vi "Live ROI Information Display.vi"(0 "Event Type":T1=enum."Value Change", 2 "ROI Mask REF":T2, 11 "IMAQ Image Display Ref":refnum<vi>) -> ()   [LabVIEW 2016]
uses:
  <vilib>/vision/Image Controls.llb/IMAQ Image.ctl
  <vilib>/event_ctls.llb/lveventtype.ctl
  Hardware Configuration/Hardware Configuration Controls/Standard Action.ctl
  <vilib>/vision/NI_Vision_Development_Module.lvlib
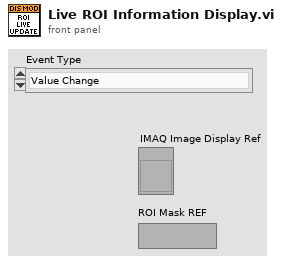
[diagram p1: front panel]
types:
  T1 = typedef "lveventtype.ctl" = enum32{"Null", "Timeout", "Annotation Menu Selection", "Annotation Menu Selection?", "App Instance Close", "App Instance Close?", "Autoscale Range Change", "Bookmark Info Change", "Cell Edit", "Cell Edit?", "Cursor Grab", "Cursor Grab?", "Cursor Menu Selection", "Cursor Menu Selection?", "Cursor Move", "Cursor Release", "Data Change", "Direction Change", "Display State Change", "Drag Ended", "Drag Enter", "Drag Leave", "Drag Over", "Drag Source Update", "Drag Starting", "Drag Starting?", "Drop", "Exec State Change", "Key Down", "Key Down?", "Key Repeat", "Key Repeat?", "Key Up", "Listbox Double Click", "Menu Activation?", "Menu Selection (App)", "Menu Selection? (App)", "Menu Selection (User)", "Mouse Down", "Mouse Down?", "Mouse Enter", "Mouse Leave", "Mouse Move", "Mouse Up", "Mouse Wheel", "NI Security User Change (App)", "Pane Size", "Panel Close", "Panel Close?", "Panel Resize", "Plot Attribute Change", "Scale Range Change", "Shortcut Menu Activation?", "Shortcut Menu Selection (App)", "Shortcut Menu Selection? (App)", "Shortcut Menu Selection (User)", "Tree Double Click", "Tree Drag", "Tree Drag?", "Tree Drop", "Tree Drop?", "Tree Item Close", "Tree Item Close?", "Tree Item Open", "Tree Item Open?", "User Event", "Value Change"}
  T2 = typedef "IMAQ Image.ctl" = refnum<image>
  T3 = typedef "Standard Action.ctl" = enum16{"Read", "Write"}
  T4 = cluster{"Global Rectangle":i32[], "Contours":cluster{"Contour Type":u32, "ROI Type":u32, "Points":i32[]}[]}
  T5 = cluster{"Contour Type":u32, "ROI Type":u32, "Points":i32[]}[]
  T6 = cluster{"Contour Type":u32, "ROI Type":u32, "Points":i32[]}
  T7 = cluster{"Mean Value":sgl, "Standard Variation":sgl, "Minimal Value":sgl, "Maximal Value":sgl, "Area (calibrated)":sgl, "Area (pixels)":u32, "%":sgl, "Calibration Valid":bool}
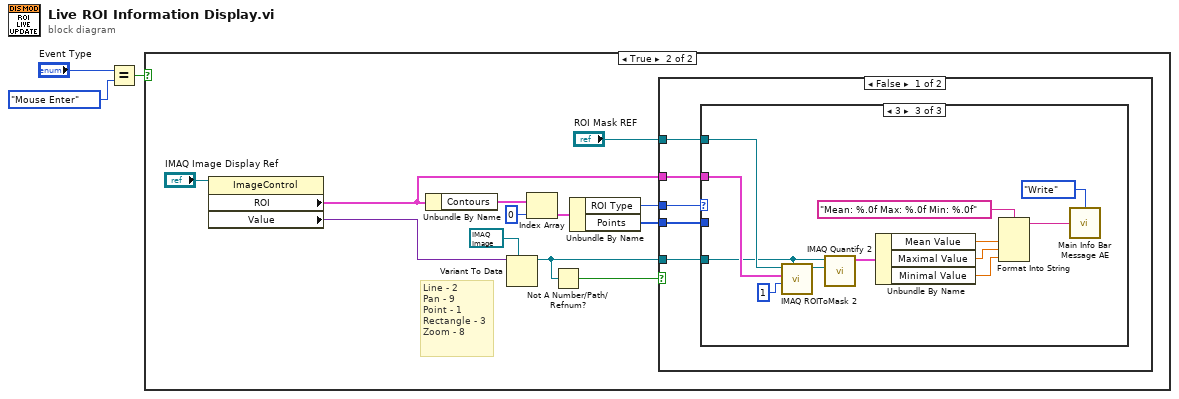
[diagram p0: block diagram]
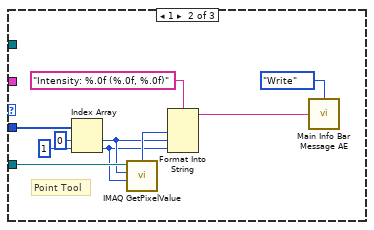
[diagram p4: hidden frame]
diagram:
  n1 = Equal?(x="Event Type", y=lveventtype."Mouse Enter") -> (x = y?=w1:bool)
  n2 = case shown="True" w1 {
    frame False {
    }
    frame True {
      # "Line - 2\nPan - 9\nPoint - 1\nRectangle - 3\nZoom - 8"
      n3 = property class="ImageControl"(reference="IMAQ Image Display Ref") -> ("ROI"=w9:T4, "Value"=w8:variant)  [unwired: 1 in, 2 out]
      n4 = Unbundle By Name(w9) -> ("Contours"=w14:T5)
      n5 = Variant To Data(type=T2 refnum ("New Image"), Variant=w8) -> (data=w6:T2)  [unwired: 1 in, 1 out]
      n6 = Index Array(array=w14, index=0) -> (element=w12:T6)
      n7 = Not A Number/Path/Refnum?(number/path/refnum=w6) -> (NaN/Path/Refnum?=w5:bool)
      n8 = Unbundle By Name(w12) -> ("ROI Type"=w11:u32, "Points"=w10:i32[])
      n9 = case shown="False" w5 {
        tunnel: w11 -> [w20 _]
        tunnel: w10 -> [w19 _]
        tunnel: w9 -> [w18 _]
        tunnel: "ROI Mask REF" -> [w17 _]
        tunnel: w6 -> [w16 _]
        frame False {
          n10 = case shown="3" w20 {
            tunnel: w19 -> [_ w30 _]
            tunnel: w18 -> [_ _ w42]
            tunnel: w17 -> [_ _ w41]
            tunnel: w16 -> [_ w26 w40]
            frame Default {
            }
            frame 1 {
              # "Point Tool"
              n11 = Index Array(array=w30, index #1=0 ("index"), index #2=1 ("index")) -> (element #1=w24:i32, element #2=w23:i32)
              n12 = call "IMAQ GetPixelValue"("Image"=w26, "X Coordinate"=w24, "Y Coordinate"=w23) -> ("Pixel Value (U16)"=w27:u16)  [unwired: 3 in, 4 out]
              n13 = Format Into String(format string="Intensity: %.0f (%.0f, %.0f)", w27, w24, w23) -> (resulting string=w22:string)  [unwired: 2 in, 1 out]
              n14 = call "Main Info Bar Message AE.vi"("Action"=Standard_Action."Write", "Message"=w22) -> ()  [unwired: 13 in, 1 out]
            }
            frame 3 {
              n15 = call "IMAQ ROIToMask 2"("Image Model"=w40, "Filling Value (255)"=1, "ROI Descriptor"=w42, "Image"=w41) -> ("Image Out"=w39:T2)  [unwired: 5 in, 2 out]
              n16 = call "IMAQ Quantify 2"("Image Mask"=w39, "Image"=w40) -> ("Global Report"=w37:T7)  [unwired: 7 in, 2 out]
              n17 = Unbundle By Name(w37) -> ("Mean Value"=w36:sgl, "Maximal Value"=w34:sgl, "Minimal Value"=w35:sgl)
              n18 = Format Into String(format string="Mean: %.0f Max: %.0f Min: %.0f", w36, w34, w35) -> (resulting string=w31:string)  [unwired: 2 in, 1 out]
              n19 = call "Main Info Bar Message AE.vi"("Action"=Standard_Action."Write", "Message"=w31) -> ()  [unwired: 13 in, 1 out]
            }
          }
        }
        frame True {
        }
      }
    }
  }
